vi "是否显示读取.vi"(4 "error in (no error)":errorcluster caption="错误输入（无错误）", 6 "Container State":T3 caption="容器状态", 7 "Display State In":T1 caption="显示状态输入") -> (0 "error out":errorcluster caption="错误输出", 2 "Value":bool caption="值", 3 "Display State Out":T1 caption="显示状态输出")   [LabVIEW 2014, in "DetecElecXControl.xctl"]
uses:
  DetecElecXControl.xctl
  <vilib>/_xctls/Container State.ctl
  <vilib>/_xctls/XControlSupport.lvlib
panel:
  # "将以下值显示控件替换为所需类型的显示控件。\n不要从连线板中删除该显示控件或其它显示控件。\n不要更改连线板模式。\n值显示控件应始终位于连线板输出端自顶部起第二个接线端。"
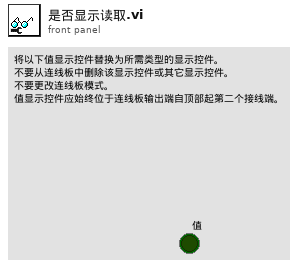
[diagram p1: front panel]
types:
  T1 = typedef "DetecElecXControl.xctl/DetecElec状态.ctl" = cluster{"是否显示":bool, "Ele":T2}
  T2 = typedef "DetecElecXControl.xctl/DetecElec数据.ctl" = cluster{"Data":bool, "ElecName":string, "mapX":string, "mapY":string, "VV":string}
  T3 = typedef "XControlSupport.lvlib/Container State.ctl" = cluster{"Indicator?":bool, "Run Mode?":bool, " Refnum":refnum<vi>}
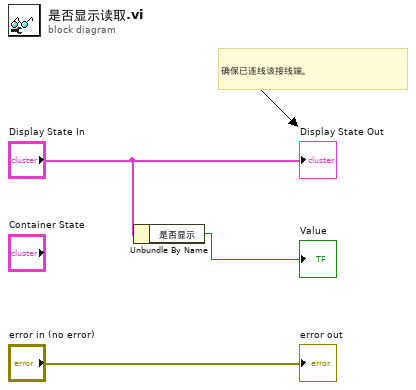
[diagram p0: block diagram]
diagram:
  # "确保已连线该接线端。"
  n1 = Unbundle By Name("Display State In") -> ("是否显示"=→"Value":bool)
  "error out" <- "error in (no error)"
  "Display State Out" <- "Display State In"
